vi "Create.vi"(8 "error in (no error)":errorcluster) -> (0 "error out":errorcluster, 3 "Pound":refnum<class "Pound.lvclass">)   [LabVIEW 2017, in "Pound.lvclass"]
doc: "Create a watchdog pound reference."
uses:
  <vilib>/NI/Software Watchdog/Pound/Pound.lvclass
  <vilib>/NI/Software Watchdog/Pound/Status.ctl
  <vilib>/NI/Software Watchdog/Pound/ExpirationType.ctl
  <vilib>/NI/Software Watchdog/Pound/Mode.ctl
  <vilib>/NI/Software Watchdog/Pound/Pound.lvclass/Pound.ctl
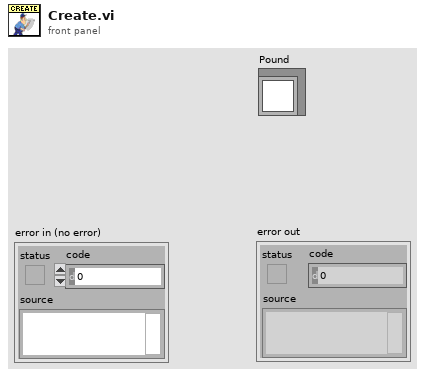
[diagram p1: front panel]
types:
  T1 = typedef "Pound.lvclass/Mode.ctl" = enum16{"Running", "Shutdown"}
  T2 = typedef "Pound.lvclass/Status.ctl" = cluster{"WatchdogName":string, "ExpirationType":T3}
  T3 = typedef "Pound.lvclass/ExpirationType.ctl" = enum16{"None", "Execution", "Shutdown"}
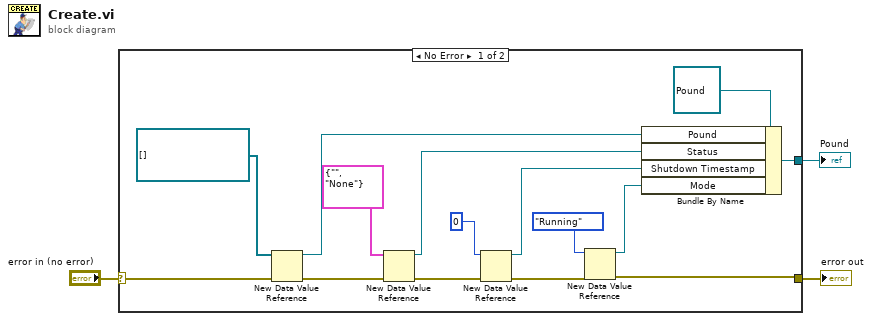
[diagram p0: block diagram]
diagram:
  n1 = case shown="No Error" "error in (no error)" {
    selector: "error in (no error)" -> [w18 w19]
    tunnel: [w8 w19] -> w2
    tunnel: [w17 _] -> w1
    frame No Error {
      n2 = New Data Value Reference(data value=refnum<data-value>[] [], error in=w18) -> (data value reference=w14:refnum<data-value>, error out=w13:errorcluster)
      n3 = New Data Value Reference(data value=T2 {"WatchdogName"="", "ExpirationType"=enum."None"} ("Status"), error in=w13) -> (data value reference=w12:refnum<data-value>, error out=w10:errorcluster)
      n4 = New Data Value Reference(data value=u32 0, error in=w10) -> (data value reference=w4:refnum<data-value>, error out=w9:errorcluster)
      n5 = New Data Value Reference(data value=Mode."Running" ("Mode"), error in=w9) -> (data value reference=w6:refnum<data-value>, error out=w8:errorcluster)
      n6 = Bundle By Name(cluster=refnum<class "Pound.lvclass"> refnum ("Pack.lvclass"), "Pound"=w14, "Status"=w12, "Shutdown Timestamp"=w4, "Mode"=w6) -> (w17:refnum<class "Pound.lvclass">)
    }
    frame Error {
    }
  }
  "error out" <- w2
  "Pound" <- w1
